vi "countrate.vi"() -> ()   [LabVIEW 2015]
uses:
  <vilib>/Platform/TimedLoop/XDataNode/timing_clust.ctl
  <vilib>/Platform/TimedLoop/XDataNode/nitl_modes.ctl
  <vilib>/Platform/TimedLoop/XDataNode/wakeup.ctl
  <vilib>/Utility/file.llb/Write Delimited Spreadsheet (I64).vi
  <vilib>/platform/TimedLoop/XDataNode/XDataNode.xnode
  <vilib>/Platform/TimedLoop/XDataNode/XDNodeRunTimeDep.lvlib
panel:
  out "Elapsed Time (s)":i64=300
  in  "File to save":path=path "C:/Users/mhsisk/week8/decay.txt"
  out "XY Graph":cluster{i64[], i32[]}(graph)={[0, 1, 2, 3, 4, 5, 6, 7, 8, 9, 10, 11, 12, 13, 14, 15, 16, 17, 18, 19, 20, 21, 22, 23, 24, 25, 26, 27, 28, 29, 30, 31, 32, 33, 34, 35, 36, 37, 38, 39, 40, 41, 42, 43, 44, 45, 46, 47, 48, 49, 50, 51, 52, 53, 54, 55, 56, 57, 58, 59, 60, 61, 62, 63, 64, 65, 66, 67, 68, 69, 70, 71, 72, 73, 74, 75, 76, 77, 78, 79, 80, 81, 82, 83, 84, 85, 86, 87, 88, 89, 90, 91, 92, 93, 94, 95, 96, 97, 98, 99, 100, 101, 102, 103, 104, 105, 106, 107, 108, 109, 110, 111, 112, 113, 114, 115, 116, 117, 118, 119, 120, 121, 122, 123, 124, 125, 126, 127, 128, 129, 130, 131, 132, 133, 134, 135, 136, 137, 138, 139, 140, 141, 142, 143, 144, 145, 146, 147, 148, 149, 150, 151, 152, 153, 154, 155, 156, 157, 158, 159, 160, 161, 162, 163, 164, 165, 166, 167, 168, 169, 170, 171, 172, 173, 174, 175, 176, 177, 178, 179, 180, 181, 182, 183, 184, 185, 186, 187, 188, 189, 190, 191, 192, 193, 194, 195, 196, 197, 198, 199, 200, 201, 202, 203, 204, 205, 206, 207, 208, 209, 210, 211, 212, 213, 214, 215, 216, 217, 218, 219, 220, 221, 222, 223, 224, 225, 226, 227, 228, 229, 230, 231, 232, 233, 234, 235, 236, 237, 238, 239, 240, 241, 242, 243, 244, 245, 246, 247, 248, 249, 250, 251, 252, 253, 254, 255, 256, 257, 258, 259, 260, 261, 262, 263, 264, 265, 266, 267, 268, 269, 270, 271, 272, 273, 274, 275, 276, 277, 278, 279, 280, 281, 282, 283, 284, 285, 286, 287, 288, 289, 290, 291, 292, 293, 294, 295, 296, 297, 298, 299, 300], [0, 61, 63, 74, 65, 56, 67, 61, 67, 57, 59, 61, 54, 70, 65, 62, 79, 61, 64, 58, 61, 68, 55, 68, 66, 55, 64, 52, 60, 38, 51, 58, 63, 53, 51, 68, 59, 41, 59, 50, 57, 55, 48, 59, 57, 68, 48, 53, 50, 64, 50, 55, 50, 55, 43, 47, 52, 47, 53, 48, 50, 56, 53, 42, 47, 47, 43, 38, 54, 47, 41, 39, 49, 44, 53, 50, 57, 41, 46, 42, 46, 27, 37, 39, 36, 34, 31, 43, 37, 32, 41, 37, 44, 36, 29, 35, 29, 45, 40, 36, 30, 54, 30, 29, 40, 27, 35, 37, 29, 30, 31, 28, 29, 26, 40, 36, 25, 32, 35, 23, 27, 25, 26, 30, 22, 27, 18, 31, 22, 28, 19, 29, 29, 21, 25, 30, 17, 27, 28, 17, 26, 16, 24, 33, 19, 25, 30, 26, 26, 18, 19, 23, 25, 25, 13, 20, 28, 18, 19, 22, 25, 13, 28, 13, 25, 20, 24, 20, 26, 18, 18, 15, 23, 20, 17, 21, 24, 26, 17, 24, 19, 19, 11, 25, 21, 14, 16, 15, 20, 15, 15, 14, 16, 14, 17, 17, 25, 17, 12, 18, 13, 20, 16, 21, 19, 12, 26, 22, 11, 8, 13, 20, 16, 17, 17, 14, 9, 12, 17, 17, 16, 12, 14, 16, 17, 15, 13, 9, 10, 12, 17, 16, 13, 10, 6, 15, 16, 8, 17, 11, 5, 18, 18, 12, 19, 18, 15, 12, 13, 10, 10, 15, 12, 8, 8, 13, 10, 14, 9, 10, 13, 11, 11, 7, 14, 11, 8, 12, 12, 10, 7, 11, 6, 10, 10, 5, 11, 6, 11, 9, 6, 8, 11, 6, 15, 7, 12, 3, 13, 8, 11, 14, 6, 9, 12, 5, 10, 11, 7, 11, 8]}
  in  "Acquisition Time (s)":i64=300
  in  "Period (s)":i64=1
  out "counts per interval":dbl(knob)=8.0 scale=0.0..100.0
  in  "stop":bool
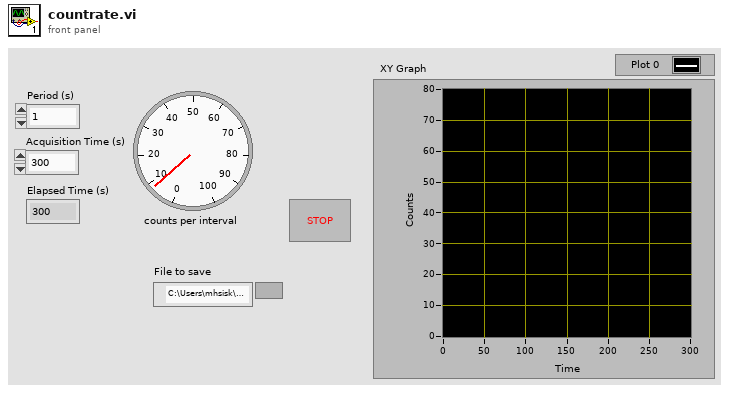
[diagram p1: front panel]
types:
  T1 = typedef "XDNodeRunTimeDep.lvlib/timing_clust.ctl" = cluster{"Expected End [f-1]":u64, "Actual End [f-1]":u64, "Finished Late? [f-1]":bool, "Expected End [i-1]":u64, "Actual End [i-1]":u64, "Finished Late? [i-1]":bool, "Expected Start [i]":u64, "Actual Start [i]":u64, "Expected Start [f]":u64, "Actual Start [f]":u64, "Source Name":string, "Structure Name":string, "Period":i64, "Deadline":i64, "Offset":i64, "Start":i64, "Priority":i32, "Timeout":i32, "Mode":T2, "Wakeup Reason":T3, "Error":errorcluster, "Source Type":string, "Secondary Source Type":string, "Global End Time":u64, "Global Start Time":u64, "Frame Duration":u64, "Iteration Duration":u64, "Assigned CPU":i32, "I/O Scan Engine Mode":u32}
  T2 = typedef "XDNodeRunTimeDep.lvlib/nitl_modes.ctl" = enum32{"No Change", "Process missed periods, maintain original phase", "Discard missed periods, maintain original phase", "Process missed periods, ignore original phase", "Discard missed periods, ignore original phase"}
  T3 = typedef "XDNodeRunTimeDep.lvlib/wakeup.ctl" = enum32{"Normal", "Aborted", "Asynchronous wakeup", "Timing source error", "Timed loop error", "Timeout"}
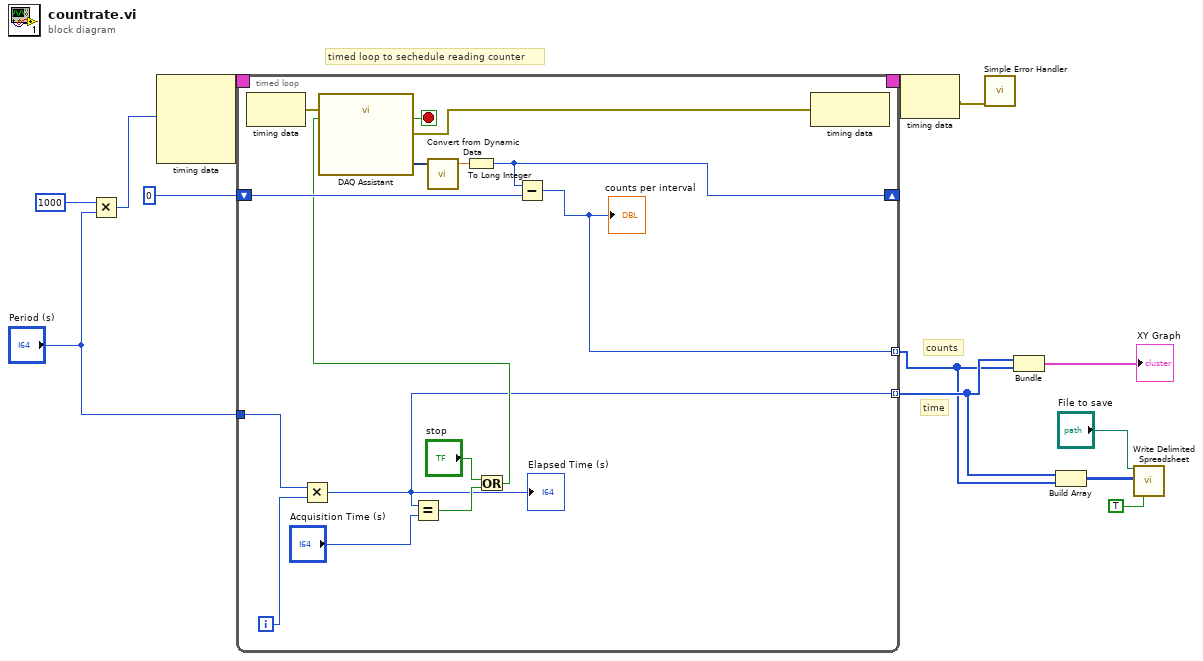
[diagram p0: block diagram]
diagram:
  # "counts"
  # "time"
  # "timed loop to sechedule reading counter"
  n1 = Multiply(x=i64 1000 ("y"), y="Period (s)") -> (x*y=w9:i64)
  n2 = node-c288(w9) -> (w13:T1)  [unwired: 3 in]
  n3 = timed-loop {
    timing: w13 -> [_]
    timing-out: [_] -> w12
    shift-right: [w18] -> _
    shift-left: 0 -> [w27]
    tunnel: "Period (s)" -> [w22]
    tunnel: [w17] -> w4 mode=indexing
    tunnel: [w16] -> w5 mode=indexing
    i -> [w15]
    stop <- w26 stop-if-true
    n4 = node-c288() -> (w23:errorcluster)  [unwired: 1 in]
    n5 = Multiply(x=w22, y=w15) -> (x*y=w16:i64)
    "Elapsed Time (s)" <- w16
    n6 = Equal?(x=w16, y="Acquisition Time (s)") -> (x = y?=w20:bool)
    n7 = Or(x="stop", y=w20) -> (x .or. y?=w19:bool)
    n8 = call "DAQ Assistant"("error in"=w23, "stop (F)"=w19) -> ("data"=w28:dynamicdata, "stopped"=w26:bool, "error out"=w24:errorcluster)  [unwired: 14 in, 1 out]
    n9 = call "Convert from Dynamic Data"("Dynamic Data Type"=w28) -> ("Scalar"=w25:dbl)  [unwired: 3 in]
    n10 = To Long Integer(number=w25) -> (32bit integer=w18:i32)
    n11 = Subtract(x=w18, y=w27) -> (x-y=w17:i32)
    "counts per interval" <- w17
    n12 = node-c288(w24) -> ()  [unwired: 1 out]
  }
  n13 = node-c288(w12) -> (w10:errorcluster)
  n14 = call <vilib>:"Simple Error Handler.vi"("error in (no error)"=w10) -> ()  [unwired: 4 in, 5 out]
  n15 = Bundle(w5, w4) -> (→"XY Graph":cluster{i64[], i32[]})  [unwired: 1 in]
  n16 = Build Array(w5, w4) -> (w3:i64[][])
  n17 = call-poly <vilib>:"Write Delimited Spreadsheet.vi"("file path (dialog if empty)"="File to save", "2D data"=w3, "transpose? (F)"=TRUE) -> ()  [unwired: 11 in, 2 out]
